vi "Write Handle.vi"(8 "error in (no error)":errorcluster, 11 "Channel in":refnum<class "Channel.lvclass">) -> (0 "error out":errorcluster, 3 "Channel out":refnum<class "Channel.lvclass">)   [LabVIEW 2018, in "Channel.lvclass"]
uses:
  Channel.lvclass
  Channel.lvclass/Channel.ctl
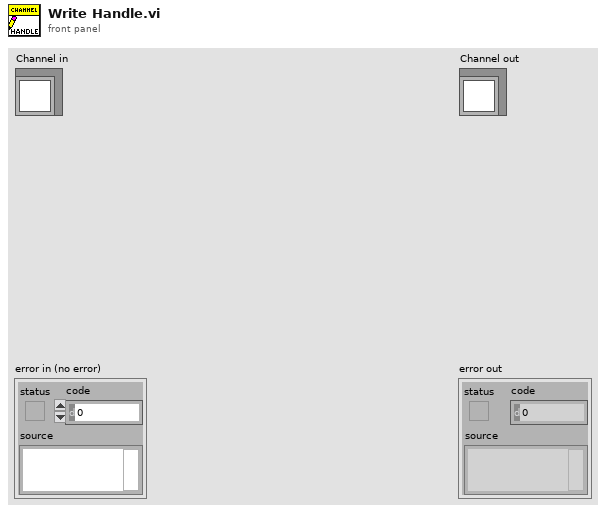
[diagram p1: front panel]
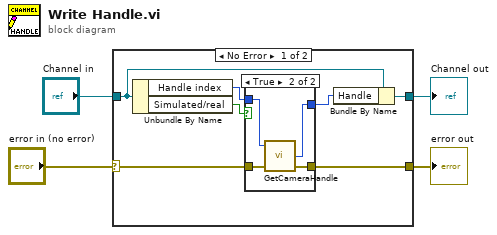
[diagram p0: block diagram]
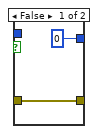
[diagram p2: hidden frame]
diagram:
  n1 = case shown="No Error" "error in (no error)" {
    selector: "error in (no error)" -> [w5 w18]
    tunnel: [w10 w18] -> w3
    tunnel: [w11 w19] -> w1
    tunnel: "Channel in" -> [w8 w19]
    frame No Error {
      n2 = Unbundle By Name(w8) -> ("Handle index"=w7:u16, "Simulated/real"=w6:bool)
      n3 = case shown="True" w6 {
        tunnel: [w12 w17] -> w10
        tunnel: [0 ("cameraHandle") w16] -> w9
        tunnel: w7 -> [_ w15]
        tunnel: w5 -> [w12 w14]
        frame False {
        }
        frame True {
          n4 = call <userlib>:"GetCameraHandle.vi"("error in (no error)"=w14, "cameraIndex"=w15) -> ("error out"=w17:errorcluster, "cameraHandle"=w16:i32)  [unwired: 1 in, 1 out]
        }
      }
      n5 = Bundle By Name(cluster=w8, "Handle"=w9) -> (w11:refnum<class "Channel.lvclass">)
    }
    frame Error {
    }
  }
  "error out" <- w3
  "Channel out" <- w1
